vi "SSCP_init.vi"(0 "config file":path=path "F:/Projects/simple-system-control-protocol/simple-system-control-protocol/source/python/lp_em_cc2340r5_example.yml", 2 "error in (no error)":errorcluster) -> (3 "Parameter Descriptors":T2[](array[typedef]), 4 "Register Descriptors":T3[](array[typedef]), 5 "Device Configuration":T1, 6 "error out":errorcluster)   [LabVIEW 2020]
uses:
  typedefs/Register Descriptor.ctl
  typedefs/Parameter Descriptor.ctl
  typedefs/Device Configuration.ctl
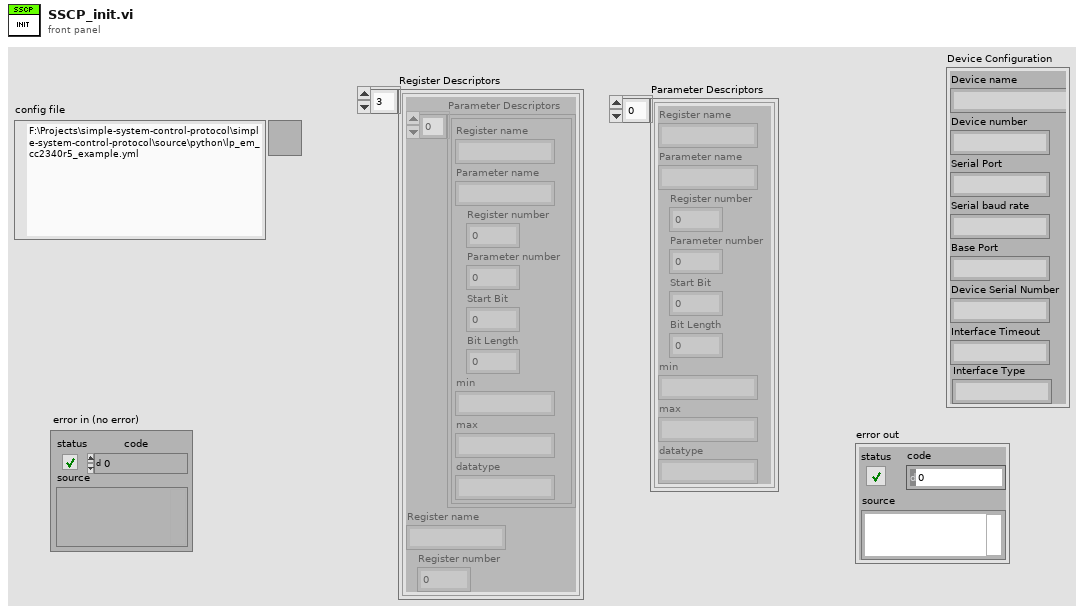
[diagram p1: front panel]
types:
  T1 = typedef "Device Configuration.ctl" = cluster{"Device name":string, "Device number":string, "Serial Port":string, "Serial baud rate":string, "Base Port":string, "Device Serial Number":string, "Interface Timeout":string, "Interface Type":string}
  T2 = typedef "Parameter Descriptor.ctl" = cluster{"Register name":string, "Parameter name":string, "Register number":i32, "Parameter number":i32, "Start Bit":i32, "Bit Length":i32, "min":string, "max":string, "datatype":string}
  T3 = typedef "Register Descriptor.ctl" = cluster{"Parameter Descriptors":T2[], "Register name":string, "Register number":i32}
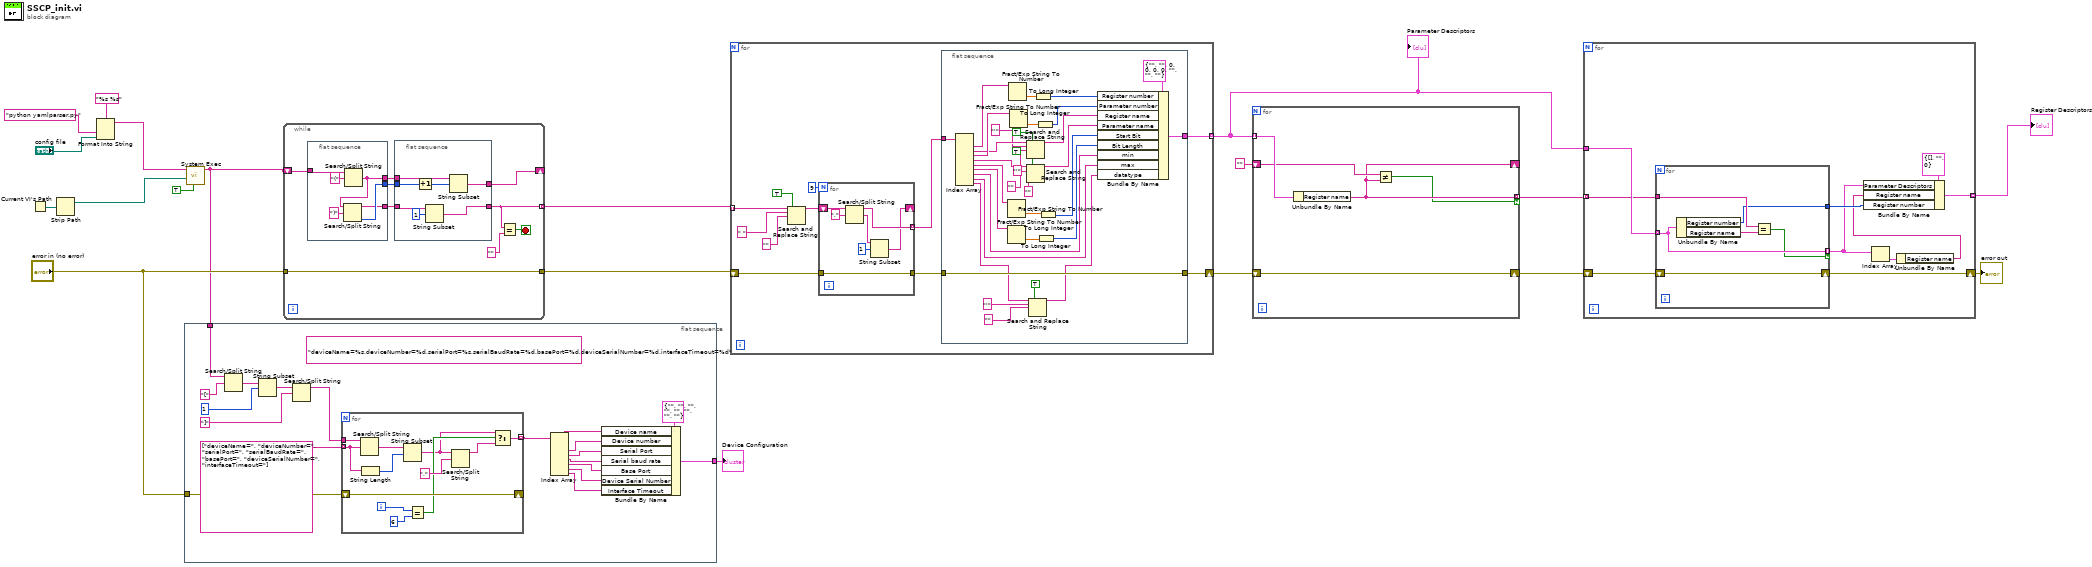
[diagram p0: block diagram]
diagram:
  n1 = Current VI's Path() -> (path=w19:path)
  n2 = Strip Path(path=w19) -> (stripped path=w14:path)  [unwired: 1 out]
  n3 = Format Into String(format string="%s %s", "python yamlparser.py", "config file") -> (resulting string=w15:string)  [unwired: 2 in, 1 out]
  n4 = flat-sequence {
    tunnel: "error in (no error)" -> [w30]
    tunnel: w2 -> [w38]
    tunnel: [w20] -> w1
    frame #0 {
      (unwired) "deviceName=%s,deviceNumber=%d,serialPort=%s,serialBaudRate=%d,basePort=%d,deviceSerialNumber=%d,interfaceTimeout=%d" ("format string")
      n5 = Search/Split String(string=w38, search string/char (-)="[") -> (match + rest of string=w35:string)  [unwired: 1 in, 2 out]
      n6 = String Subset(string=w35, offset (0)=1) -> (substring=w33:string)  [unwired: 1 in]
      n7 = Search/Split String(string=w33, search string/char (-)="]") -> (substring before match=w32:string)  [unwired: 1 in, 2 out]
      n8 = for {
        tunnel: w32 -> [w50]
        tunnel: string[] ["deviceName=", "deviceNumber=", "serialPort=", "serialBaudRate=", "basePort=", "deviceSerialNumber=", "interfaceTimeout="] -> [w46] mode=indexing
        shift-right: [w45] -> _
        shift-left: w30 -> [w45]
        tunnel: [w39] -> w29 mode=indexing
        i -> [w44]
        n9 = Search/Split String(string=w50, search string/char (-)=w46) -> (match + rest of string=w49:string)  [unwired: 1 in, 2 out]
        n10 = String Length(string=w46) -> (length=w48:i32)
        n11 = String Subset(string=w49, offset (0)=w48) -> (substring=w40:string)  [unwired: 1 in]
        n12 = Equal?(x=w44, y=6) -> (x = y?=w42:bool)
        n13 = Search/Split String(string=w40, search string/char (-)=",") -> (substring before match=w41:string)  [unwired: 1 in, 2 out]
        n14 = Select(t=w40, s=w42, f=w41) -> (s? t:f=w39:string)
      }
      n15 = Index Array(array=w29) -> (element #1=w27:string, element #2=w26:string, element #3=w25:string, element #4=w24:string, element #5=w23:string, element #6=w22:string, element #7=w21:string)  [unwired: 7 in]
      n16 = Bundle By Name(cluster=T1 {"Device name"="", "Device number"="", "Serial Port"="", "Serial baud rate"="", "Base Port"="", "Device Serial Number"="", "Interface Timeout"="", "Interface Type"=""} ("Device Configuration"), "Device name"=w27, "Device number"=w26, "Serial Port"=w25, "Serial baud rate"=w24, "Base Port"=w23, "Device Serial Number"=w22, "Interface Timeout"=w21) -> (w20:T1)
    }
  }
  n17 = call <vilib>:"System Exec.vi"("run minimized? (F)"=TRUE, "working directory"=w14, "command line"=w15) -> ("standard output"=w2:string)  [unwired: 5 in, 3 out]
  n18 = while {
    shift-right: [w56] -> _
    shift-left: w2 -> [w59]
    tunnel: [w53] -> w12 mode=indexing
    tunnel: "error in (no error)" -> [w51]
    tunnel: [w51] -> w11
    stop <- w54 stop-if-true
    n19 = flat-sequence {
      tunnel: w59 -> [w71]
      tunnel: [w67] -> w58
      tunnel: [w69] -> w57
      tunnel: [w68] -> w55
      frame #0 {
        n20 = Search/Split String(string=w71, search string/char (-)="(") -> (match + rest of string=w67:string)  [unwired: 1 in, 2 out]
        n21 = Search/Split String(string=w67, search string/char (-)=")") -> (substring before match=w68:string, offset of match=w69:i32)  [unwired: 1 in, 1 out]
      }
    }
    n22 = flat-sequence {
      tunnel: w58 -> [w66]
      tunnel: w57 -> [w65]
      tunnel: [w63] -> w56
      tunnel: w55 -> [w62]
      tunnel: [w61] -> w53
      frame #0 {
        n23 = Increment(x=w65) -> (x+1=w64:i32)
        n24 = String Subset(string=w62, offset (0)=1) -> (substring=w61:string)  [unwired: 1 in]
        n25 = String Subset(string=w66, offset (0)=w64) -> (substring=w63:string)  [unwired: 1 in]
      }
    }
    n26 = Equal?(x=w53, y="") -> (x = y?=w54:bool)
  }
  n27 = for {
    tunnel: w12 -> [w83] mode=indexing
    tunnel: [w75] -> w6 mode=indexing
    shift-right: [w73] -> w10
    shift-left: w11 -> [w77]
    n28 = Search and Replace String(replace all?=TRUE ("replace all? (F)"), input string=w83, search string=" ", replace string="" ("replace string (\"\")")) -> (result string=w78:string)  [unwired: 4 in, 3 out]
    n29 = for {
      N: 9 -> [_]
      shift-right: [w117] -> _
      shift-left: w78 -> [w123]
      tunnel: [w121] -> w76 mode=indexing
      tunnel: w77 -> [w120]
      tunnel: [w120] -> w74
      n30 = Search/Split String(string=w123, search string/char (-)=",") -> (substring before match=w121:string, match + rest of string=w119:string)  [unwired: 1 in, 1 out]
      n31 = String Subset(string=w119, offset (0)=1) -> (substring=w117:string)  [unwired: 1 in]
    }
    n32 = flat-sequence {
      tunnel: w76 -> [w116]
      tunnel: [w100] -> w75
      tunnel: w74 -> [w99]
      tunnel: [w99] -> w73
      frame #0 {
        n33 = Index Array(array=w116) -> (element #1=w114:string, element #2=w98:string, element #3=w111:string, element #4=w94:string, element #5=w108:string, element #6=w105:string, element #7=w102:string, element #8=w101:string, element #9=w85:string)  [unwired: 9 in]
        n34 = Fract/Exp String To Number(string=w108) -> (number=w107:dbl)  [unwired: 3 in, 1 out]
        n35 = Fract/Exp String To Number(string=w105) -> (number=w104:dbl)  [unwired: 3 in, 1 out]
        n36 = Fract/Exp String To Number(string=w114) -> (number=w113:dbl)  [unwired: 3 in, 1 out]
        n37 = Fract/Exp String To Number(string=w111) -> (number=w110:dbl)  [unwired: 3 in, 1 out]
        n38 = Search and Replace String(replace all?=TRUE ("replace all? (F)"), input string=w98, search string="'", replace string="" ("replace string (\"\")")) -> (result string=w96:string)  [unwired: 4 in, 3 out]
        n39 = Search and Replace String(replace all?=TRUE ("replace all? (F)"), input string=w94, search string="'", replace string="" ("replace string (\"\")")) -> (result string=w93:string)  [unwired: 4 in, 3 out]
        n40 = Search and Replace String(replace all?=TRUE ("replace all? (F)"), input string=w85, search string="'", replace string="" ("replace string (\"\")")) -> (result string=w84:string)  [unwired: 4 in, 3 out]
        n41 = To Long Integer(number=w113) -> (32bit integer=w112:i32)
        n42 = To Long Integer(number=w110) -> (32bit integer=w109:i32)
        n43 = To Long Integer(number=w104) -> (32bit integer=w103:i32)
        n44 = To Long Integer(number=w107) -> (32bit integer=w106:i32)
        n45 = Bundle By Name(cluster=T2 {"Register name"="", "Parameter name"="", "Register number"=0, "Parameter number"=0, "Start Bit"=0, "Bit Length"=0, "min"="", "max"="", "datatype"=""} ("Cluster"), "Register number"=w112, "Parameter number"=w109, "Register name"=w96, "Parameter name"=w93, "Start Bit"=w106, "Bit Length"=w103, "min"=w102, "max"=w101, "datatype"=w84) -> (w100:T2)
      }
    }
  }
  "Parameter Descriptors" <- w6
  n46 = for {
    shift-right: [w124] -> w8
    shift-left: w10 -> [w124]
    tunnel: w6 -> [w128] mode=indexing
    shift-right: [w126] -> _
    shift-left: "" -> [w127]
    tunnel: [w126] -> w7 mode=indexing if=w125
    n47 = Unbundle By Name(w128) -> ("Register name"=w126:string)
    n48 = Not Equal?(x=w127, y=w126) -> (x != y?=w125:bool)
  }
  n49 = for {
    shift-right: [w137] -> w4
    shift-left: w8 -> [w138]
    tunnel: w7 -> [w135] mode=indexing
    tunnel: w6 -> [w136]
    tunnel: [w132] -> w5 mode=indexing
    n50 = for {
      shift-right: [w144] -> w137
      shift-left: w138 -> [w144]
      tunnel: w136 -> [w142] mode=indexing
      tunnel: w135 -> [w143]
      tunnel: [w142] -> w131 mode=indexing if=w141
      tunnel: [w139] -> w133
      n51 = Unbundle By Name(w142) -> ("Register number"=w139:i32, "Register name"=w140:string)
      n52 = Equal?(x=w143, y=w140) -> (x = y?=w141:bool)
    }
    n53 = Index Array(array=w131) -> (element=w130:T2)  [unwired: 1 in]
    n54 = Unbundle By Name(w130) -> ("Register name"=w129:string)
    n55 = Bundle By Name(cluster=T3 {"Parameter Descriptors"=[], "Register name"="", "Register number"=0} ("Register Descriptor"), "Parameter Descriptors"=w131, "Register name"=w129, "Register number"=w133) -> (w132:T3)
  }
  "Register Descriptors" <- w5
  "error out" <- w4
  "Device Configuration" <- w1
